vi "TCP Client Test.vi"() -> ()   [LabVIEW 2019]
panel:
  out "command line":string="shutdown -P -h now"
  out "Loop index":i32
  in  "bytes to read":i32
  in  "timeout ms (25000)":i32
  out "Server message":string
  out "In Read Loop":bool
  in  "Stop":bool
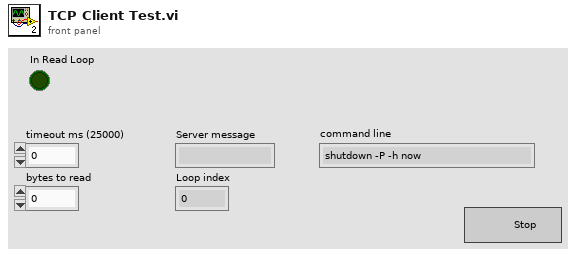
[diagram p1: front panel]
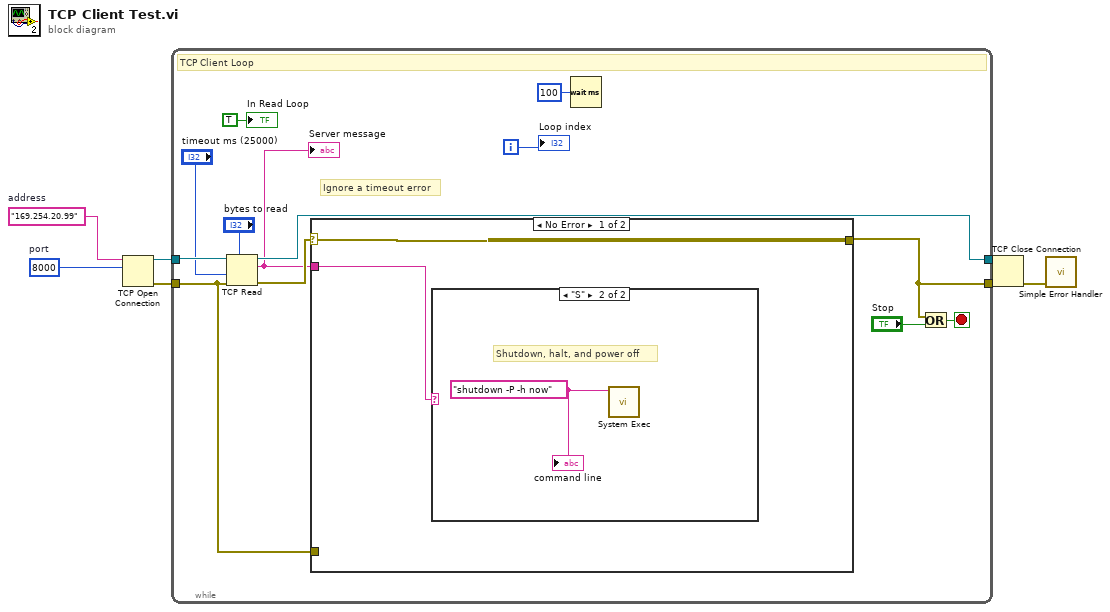
[diagram p0: block diagram]
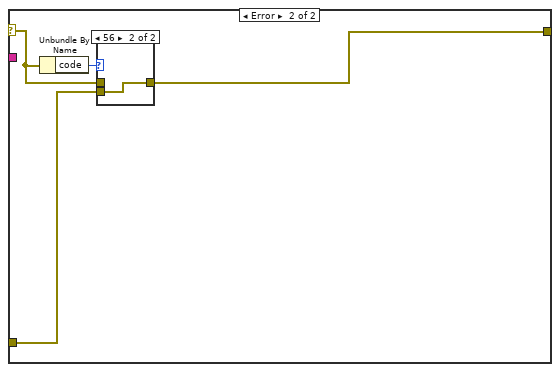
[diagram p3: hidden frame]
diagram:
  w4 = u16 8000  # port
  w5 = "169.254.20.99"  # address
  n1 = TCP Open Connection(address=w5, remote port or service name=w4) -> (connection ID=w7:refnum<k5>, error out=w6:errorcluster)  [unwired: 3 in]
  n2 = while {
    tunnel: w6 -> [w11]
    tunnel: w7 -> [w17]
    tunnel: [w10] -> w2
    tunnel: [w9] -> w1
    i -> [w15]
    stop <- w19 stop-if-true
    # "Ignore a timeout error"
    # "TCP Client Loop"
    n3 = TCP Read(connection ID=w17, bytes to read="bytes to read", error in (no error)=w11, 9:"timeout ms (25000)") -> (connection ID out=w9:refnum<k5>, data out=w8:string, error out=w12:errorcluster)  [unwired: 1 in]
    "Server message" <- w8
    n4 = case shown="No Error" w12 {
      selector: w12 -> [w22 w26]
      tunnel: [w22 w24] -> w10
      tunnel: w11 -> [_ w25]
      tunnel: w8 -> [w21 _]
      frame No Error {
        n5 = case shown="\"S\"" w21 {
          frame "False", Default {
          }
          frame "S" {
            w23 = "shutdown -P -h now" ("command line")
            # "Shutdown, halt, and power off"
            n6 = call <vilib>:"System Exec.vi"("command line"=w23) -> ()  [unwired: 7 in, 4 out]
            "command line" <- w23
          }
        }
      }
      frame Error {
        n7 = Unbundle By Name(w26) -> ("code"=w27:i32)
        n8 = case shown="56" w27 {
          tunnel: w26 -> [w28 _]
          tunnel: w25 -> [_ w29]
          tunnel: [w28 w29] -> w24
          frame Default {
          }
          frame 56 {
          }
        }
      }
    }
    n9 = Wait (ms)(milliseconds to wait=u32 100) -> ()  [unwired: 1 out]
    n10 = Or(x=w10, y="Stop") -> (x .or. y?=w19:bool)
    "In Read Loop" <- TRUE ("In Read Loop")
    "Loop index" <- w15
  }
  n11 = TCP Close Connection(connection ID=w1, error in (no error)=w2) -> (error out=w3:errorcluster)  [unwired: 1 in, 1 out]
  n12 = call <vilib>:"Simple Error Handler.vi"("error in (no error)"=w3) -> ()  [unwired: 4 in, 5 out]
